vi "Operator Joystick.vi"(9 "Buttons":bool[](array[boolean]), 10 "Axes":dbl[](array[numeric])) -> ()   [LabVIEW 2018]
panel:
  out "Intake Wrist":T1(ring)
  out "Elevator Level":T2(ring)
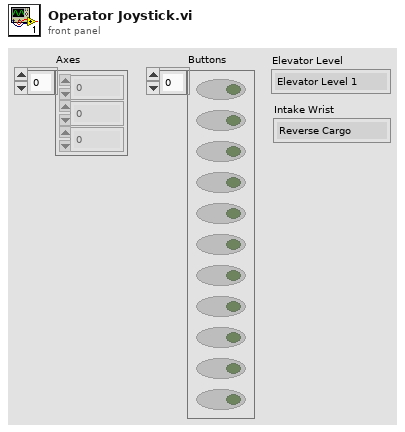
[diagram p1: front panel]
types:
  T1 = enum16{"Reverse Cargo", "Outtake Cargo", "Intake Cargo", "Outtake Hatches", "Intake Hatches"}
  T2 = enum16{"Elevator Level 1", "Elevator Level 2", "Elevator Level 3"}
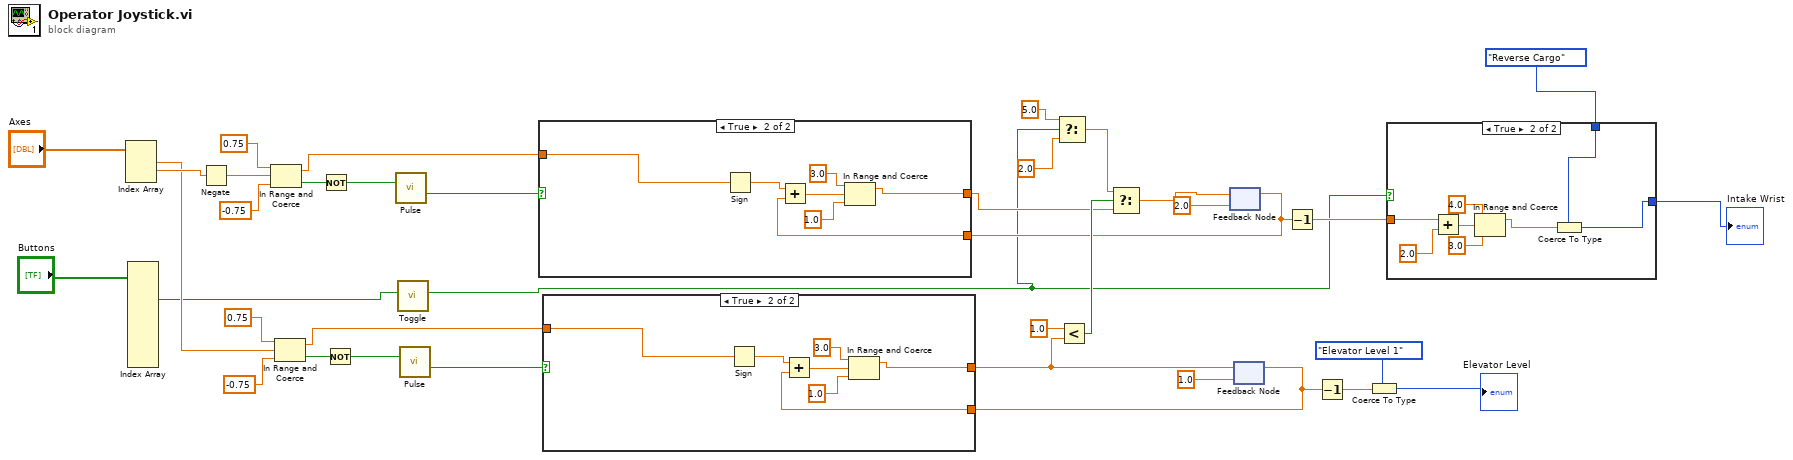
[diagram p0: block diagram]
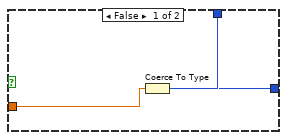
[diagram p2: hidden frame]
diagram:
  n1 = Index Array(array="Axes") -> (element #1=w19:dbl, element #2=w28:dbl)  [unwired: 3 in, 1 out]
  n2 = Index Array(array="Buttons") -> (element #3=w8:bool)  [unwired: 11 in, 10 out]
  n3 = Negate(x=w28) -> (-x=w27:dbl)
  n4 = In Range and Coerce(upper limit=0.75, x=w27, lower limit=-0.75) -> (coerced(x)=w33:dbl, In Range?=w29:bool)
  n5 = In Range and Coerce(upper limit=0.75, x=w19, lower limit=-0.75) -> (coerced(x)=w22:dbl, In Range?=w26:bool)
  n6 = Not(x=w29) -> (.not. x?=w31:bool)
  n7 = Not(x=w26) -> (.not. x?=w24:bool)
  n8 = call "Pulse.vi"("Input"=w31) -> ("Output"=w30:bool)  [unwired: 10 in]
  n9 = call "Toggle.vi"("Input"=w8) -> ("Output"=w1:bool)  [unwired: 10 in]
  n10 = call "Pulse.vi"("Input"=w24) -> ("Output"=w25:bool)  [unwired: 10 in]
  n11 = Select(t=5.0, s=w1, f=2.0) -> (s? t:f=w2:dbl)
  n12 = feedback #1(2.0) -> (w13:dbl)
  n13 = case shown="True" w30 {
    tunnel: w33 -> [_ w45]
    tunnel: [w38 w39] -> w15
    tunnel: w13 -> [w38 w44]
    frame False {
    }
    frame True {
      n14 = Sign(1:w45) -> (0:w43:dbl)
      n15 = Add(x=w43, y=w44) -> (x+y=w42:dbl)
      n16 = In Range and Coerce(upper limit=3.0, x=w42, lower limit=1.0) -> (coerced(x)=w39:dbl)  [unwired: 1 out]
    }
  }
  n17 = feedback #2(1.0) -> (w12:dbl)
  n18 = case shown="True" w25 {
    tunnel: w22 -> [_ w53]
    tunnel: [w46 w47] -> w18
    tunnel: w12 -> [w46 w52]
    frame False {
    }
    frame True {
      n19 = Sign(1:w53) -> (0:w51:dbl)
      n20 = Add(x=w51, y=w52) -> (x+y=w50:dbl)
      n21 = In Range and Coerce(upper limit=3.0, x=w50, lower limit=1.0) -> (coerced(x)=w47:dbl)  [unwired: 1 out]
    }
  }
  n22 = Less?(x=1.0, y=w18) -> (x < y?=w16:bool)
  n23 = Select(t=w2, s=w16, f=w15) -> (s? t:f=w14:dbl)
  n24 = feedback-in #1(w14) -> ()
  n25 = feedback-in #2(w18) -> ()
  n26 = Decrement(x=w13) -> (x-1=w6:dbl)
  n27 = Decrement(x=w12) -> (x-1=w11:dbl)
  n28 = Coerce To Type(0:w11, 1:T2."Elevator Level 1") -> (2:→"Elevator Level":T2)
  n29 = case shown="True" w1 {
    tunnel: T1."Reverse Cargo" -> [w56 w64]
    tunnel: w6 -> [w55 w63]
    tunnel: [w54 w60] -> w5
    frame False {
      n30 = Coerce To Type(0:w55, 1:w56) -> (2:w54:T1)
    }
    frame True {
      n31 = Add(x=w63, y=2.0 ("x")) -> (x+y=w59:dbl)
      n32 = In Range and Coerce(upper limit=4.0, x=w59, lower limit=3.0) -> (coerced(x)=w61:dbl)  [unwired: 1 out]
      n33 = Coerce To Type(0:w61, 1:w64) -> (2:w60:T1)
    }
  }
  "Intake Wrist" <- w5
